vi "9.4.-SubVI Distancias Centroide a Contorno.vi"(9 "Yc":dbl, 10 "Xc":dbl, 11 "Array in":u32[][](array[numeric])) -> (1 "Distancias 2":dbl[](array[numeric]), 2 "Distancias":dbl[](array[numeric]), 3 "Firma de la imagen":cluster{i32[], dbl[]}(graph))   [LabVIEW 2020]
panel:
  # "Visión Artificial - Firma de Figuras\nDiego Cervantes Rodríguez\ndicer0.com"
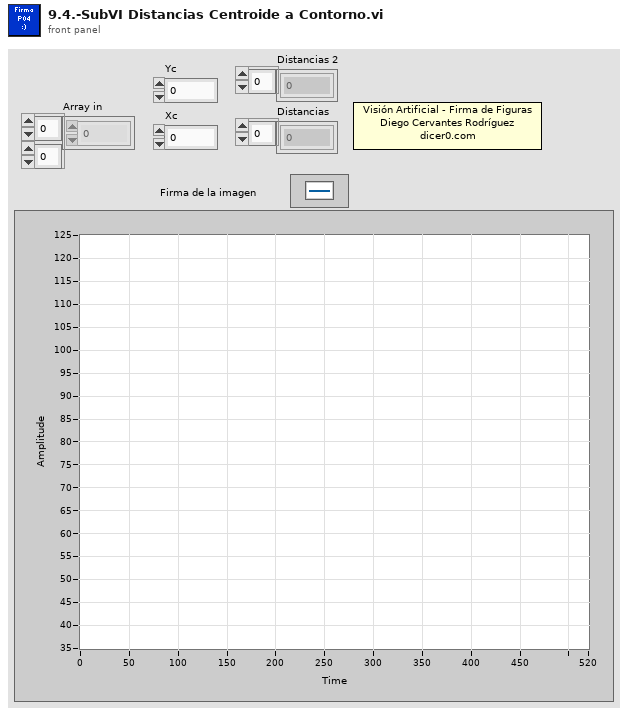
[diagram p1: front panel]
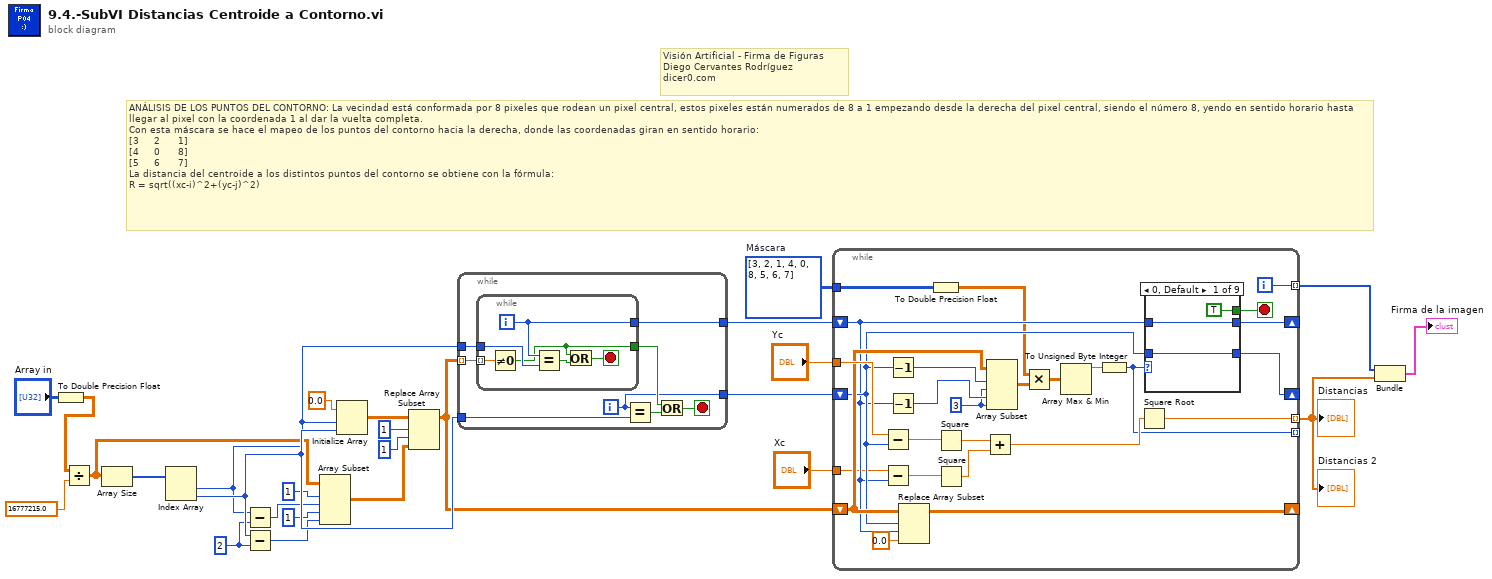
[diagram p0: block diagram]
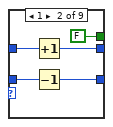
[diagram p2: hidden frame]
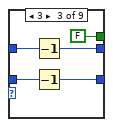
[diagram p3: hidden frame]
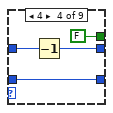
[diagram p4: hidden frame]
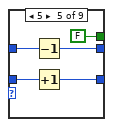
[diagram p5: hidden frame]
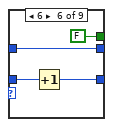
[diagram p6: hidden frame]
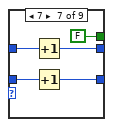
[diagram p7: hidden frame]
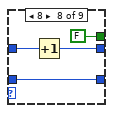
[diagram p8: hidden frame]
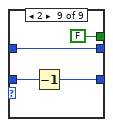
[diagram p9: hidden frame]
diagram:
  w11 = 2 ("y")
  w4 = i32[][] [[3, 2, 1], [4, 0, 8], [5, 6, 7]]  # Máscara
  # "Visión Artificial - Firma de Figuras\nDiego Cervantes Rodríguez\ndicer0.com"
  # "ANÁLISIS DE LOS PUNTOS DEL CONTORNO: La vecindad está conformada por 8 pixeles que rodean un pixel central, estos pixeles están numerados de 8 a 1 empezando desde la derecha del pixel central, siendo el número 8, yendo en sentido horario hasta llegar al pixel con la coordenada 1 al dar la vuelta completa.\nCon esta máscara se hace el mapeo de los puntos del contorno hacia la derecha, donde las coordenadas giran en sentido horario:\n[3     2      1]\n[4     0      8]\n[5     6      7]\nLa distancia del centroide a los distintos puntos del contorno se obtiene con la fórmula:\nR = sqrt((xc-i)^2+(yc-j)^2)"
  n1 = To Double Precision Float(number="Array in") -> (double precision float=w1:dbl[][])
  n2 = Divide(x=w1, y=16777215.0) -> (x/y=w16:dbl[][])
  n3 = Array Size(array=w16) -> (size(s)=w5:i32[])
  n4 = Index Array "Index Array"(array=w5) -> (element #1=w18:i32, element #2=w19:i32)  [unwired: 2 in]
  n5 = Subtract(x=w18, y=w11) -> (x-y=w10:i32)
  n6 = Subtract(x=w19, y=w11) -> (x-y=w17:i32)
  n7 = Array Subset "Array Subset"(array=w16, index (row)=1 ("index"), length (row)=w10, index (col)=1 ("index"), length (col)=w17) -> (w14:dbl[][])
  n8 = Initialize Array "Initialize Array"(0.0 ("element"), w18, w19) -> (w13:dbl[][])
  n9 = Replace Array Subset(array=w13, new element=w14, index (row)=1, index (col)=1) -> (w15:dbl[][])
  n10 = while {
    tunnel: w15 -> [w34] mode=indexing
    tunnel: [w33] -> w21
    tunnel: [w28] -> w20
    tunnel: w18 -> [w32]
    tunnel: w19 -> [w27]
    i -> [w28]
    stop <- w30 stop-if-true
    n11 = while {
      tunnel: w34 -> [w40] mode=indexing
      tunnel: [w37] -> w33
      tunnel: w32 -> [w36]
      tunnel: [w35] -> w31
      i -> [w37]
      stop <- w39 stop-if-true
      n12 = Not Equal To 0?(x=w40) -> (x != 0?=w35:bool)
      n13 = Equal?(x=w37, y=w36) -> (x = y?=w38:bool)
      n14 = Or(x=w35, y=w38) -> (x .or. y?=w39:bool)
    }
    n15 = Equal?(x=w28, y=w27) -> (x = y?=w29:bool)
    n16 = Or(x=w31, y=w29) -> (x .or. y?=w30:bool)
  }
  n17 = while {
    shift-right: [w60] -> _
    shift-left: w20 -> [w49]
    shift-right: [w59] -> _
    shift-left: w21 -> [w48]
    tunnel: w4 -> [w42]
    tunnel: "Yc" -> [w57]
    tunnel: "Xc" -> [w45]
    tunnel: [w51] -> w26 mode=indexing
    shift-right: [w46] -> _
    shift-left: w15 -> [w50]
    tunnel: [w44] -> _ mode=indexing
    tunnel: [w43] -> w22 mode=indexing
    i -> [w43]
    stop <- w58 stop-if-true
    w64 = 3 ("length")
    n18 = Subtract(x=w57, y=w49) -> (x-y=w56:dbl)
    n19 = Subtract(x=w45, y=w48) -> (x-y=w54:dbl)
    n20 = Decrement(x=w49) -> (x-1=w66:i32)
    n21 = Decrement(x=w48) -> (x-1=w65:i32)
    n22 = Replace Array Subset "Replace Array Subset"(array=w50, new element=0.0 ("new element/subarray"), index (row)=w49, index (col)=w48) -> (w46:dbl[][])
    n23 = To Double Precision Float(number=w42) -> (double precision float=w41:dbl[][])
    n24 = Square(x=w56) -> (x^2=w55:dbl)
    n25 = Square(x=w54) -> (x^2=w53:dbl)
    n26 = Add(x=w55, y=w53) -> (x+y=w52:dbl)
    n27 = Array Subset(array=w50, index (row)=w66, length (row)=w64, index (col)=w65, length (col)=w64) -> (w63:dbl[][])
    n28 = Multiply(x=w41, y=w63) -> (x*y=w62:dbl[][])
    n29 = Array Max & Min(array=w62) -> (max value=w61:dbl)  [unwired: 3 out]
    n30 = To Unsigned Byte Integer(number=w61) -> (unsigned 8bit integer=w44:u8)
    n31 = Square Root(x=w52) -> (sqrt(x)=w51:dbl)
    n32 = case shown="0, Default" w44 {
      tunnel: w49 -> [w68 w74 w79 w81 w86 w92 w97 w99 w105]
      tunnel: w48 -> [w67 w73 w77 w83 w88 w90 w95 w101 w103]
      tunnel: [w68 w72 w78 w81 w85 w91 w96 w99 w104] -> w60
      tunnel: [w67 w71 w76 w82 w87 w90 w94 w100 w103] -> w59
      tunnel: [TRUE FALSE FALSE FALSE FALSE FALSE FALSE FALSE FALSE] -> w58
      frame 0, Default {
      }
      frame 1 {
        n33 = Increment(x=w73) -> (x+1=w71:i32)
        n34 = Decrement(x=w74) -> (x-1=w72:i32)
      }
      frame 3 {
        n35 = Decrement(x=w77) -> (x-1=w76:i32)
        n36 = Decrement(x=w79) -> (x-1=w78:i32)
      }
      frame 4 {
        n37 = Decrement(x=w83) -> (x-1=w82:i32)
      }
      frame 5 {
        n38 = Decrement(x=w88) -> (x-1=w87:i32)
        n39 = Increment(x=w86) -> (x+1=w85:i32)
      }
      frame 6 {
        n40 = Increment(x=w92) -> (x+1=w91:i32)
      }
      frame 7 {
        n41 = Increment(x=w95) -> (x+1=w94:i32)
        n42 = Increment(x=w97) -> (x+1=w96:i32)
      }
      frame 8 {
        n43 = Increment(x=w101) -> (x+1=w100:i32)
      }
      frame 2 {
        n44 = Decrement(x=w105) -> (x-1=w104:i32)
      }
    }
  }
  "Distancias" <- w26
  "Distancias 2" <- w26
  n45 = Bundle "Bundle"(w22, w26) -> (→"Firma de la imagen":cluster{i32[], dbl[]})  [unwired: 1 in]
